vi "Robot Global Data.vi"() -> ()   [LabVIEW 2020]
doc: "This global VI can contain as many global variables as you need. To create a global variable, place a control on the panel, give it a good name. To read or write to it from a VI, drag the icon to the diagram of that VI. You can also drag from the project. Click on the node to change which global you access. You shouldn't have multiple locations writing to a global or it will cause a race-condition."
uses:
  <vilib>/Rock Robotics/WPI/Camera/WPI_CameraImageSize.ctl
  <vilib>/Rock Robotics/WPI/DriverStation/WPI_DriverStationRobotMode2.ctl
panel:
  in  "Intake Sped Up Duration":dbl
  in  "Intake Sped Up Setpoint":dbl
  in  "Pivot Duration":dbl
  in  "Pivot Right Speed":dbl
  in  "Pivot Left Speed":dbl
  in  "Spring Arm Setpoint":dbl
  in  "Climb Setpoint":dbl
  in  "Transfer Release Duration":dbl
  in  "Transfer Up Duration":dbl
  in  "Intake Duration":dbl
  in  "Shooter Duration":dbl
  in  "Auto Pickup":string
  in  "Auto List":string
  in  "Op Button 11":bool
  in  "Op Button 10":bool
  in  "Op Button 9":bool
  in  "Op Button 8":bool
  in  "Spring Arm":bool
  in  "Button 11":bool
  in  "Button 10":bool
  in  "Button 9":bool
  in  "Button 8":bool
  in  "Button 7":bool
  in  "Button 6":bool
  in  "Button 5":bool
  in  "Button 4":bool
  in  "Record Path Stop RB":bool
  in  "Record Path Start LB":bool
  in  "Pivot Right RT":bool
  in  "Pivot Left LT":bool
  in  "Transfer Release Setpoint":dbl
  in  "Transfer Up Setpoint":dbl
  in  "Intake Setpoint":dbl
  in  "Shooter Setpoint":dbl
  in  "Record Path":bool
  in  "Wheel":dbl
  in  "Throtle":dbl
  in  "Climb Traversal":bool
  in  "Transfer Release":bool
  in  "Transfer Up":bool
  in  "Intake Arm Down LT":bool
  in  "Intake Arm Up LB":bool
  in  "Intake RT":bool
  in  "Shooter RB":bool
  in  "Robot Mode":T1
  in  "image size":T2=enum."320x240"
  in  "Enable Vision":bool
  # "Driver Joystick Variables"
  # "Operator Joystick Variables"
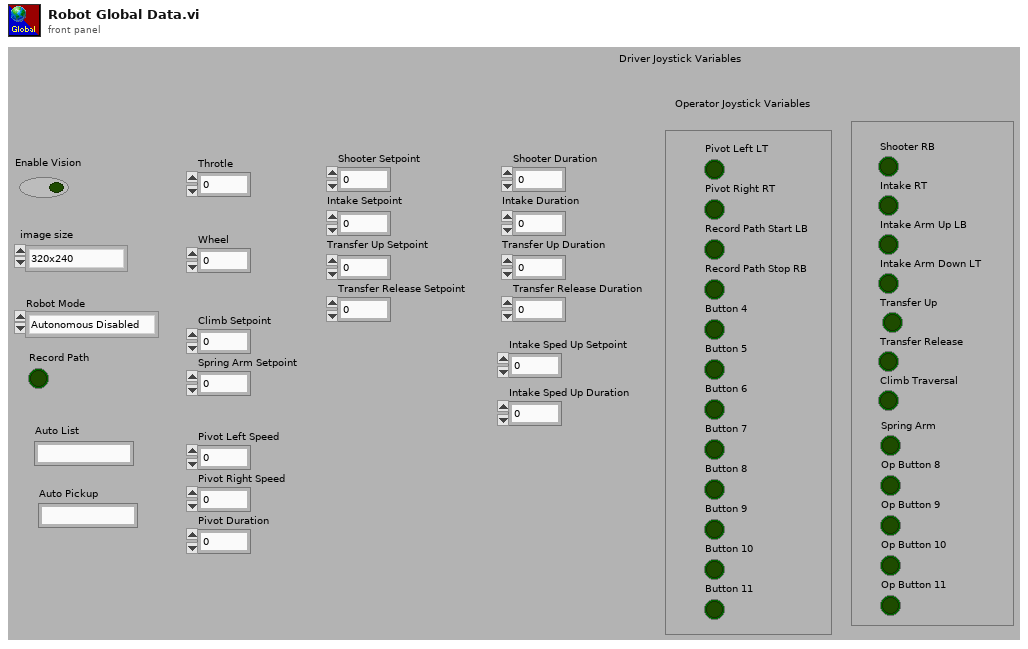
[diagram p1: front panel]
types:
  T1 = typedef "WPI_DriverStationRobotMode2.ctl" = enum16{"Autonomous Disabled", "Autonomous Enabled", "Teleop Disabled", "Teleop Enabled", "Disconnected", "Finish", "Test Disabled", "Test Enabled", "Emergency Stopped"}
  T2 = typedef "WPI_CameraImageSize.ctl" = enum16{"640x480", "320x240", "160x120", "Custom"}
diagram:
